vi "plusminus.vi"(5 "y":dbl, 6 "x":dbl) -> (1 "x - y":dbl, 2 "x + y":dbl)   [LabVIEW 2017]
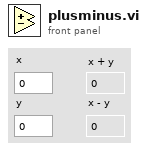
[diagram p1: front panel]
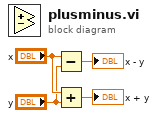
[diagram p0: block diagram]
diagram:
  n1 = Subtract(x="x", y="y") -> (x-y=→"x - y":dbl)
  n2 = Add(x="x", y="y") -> (x+y=→"x + y":dbl)
